vi "运维调试.vi"() -> ()   [LabVIEW 2016]
uses:
  <vilib>/Utility/miscctls.llb/LVPointTypeDef.ctl
  PLC/PLC.lvlib
  API/CodCr/CodCr.lvlib
  <vilib>/Utility/config.llb/NI_LVConfig.lvlib
panel:
  in  "运维调试菜单":T1(xcontrol)
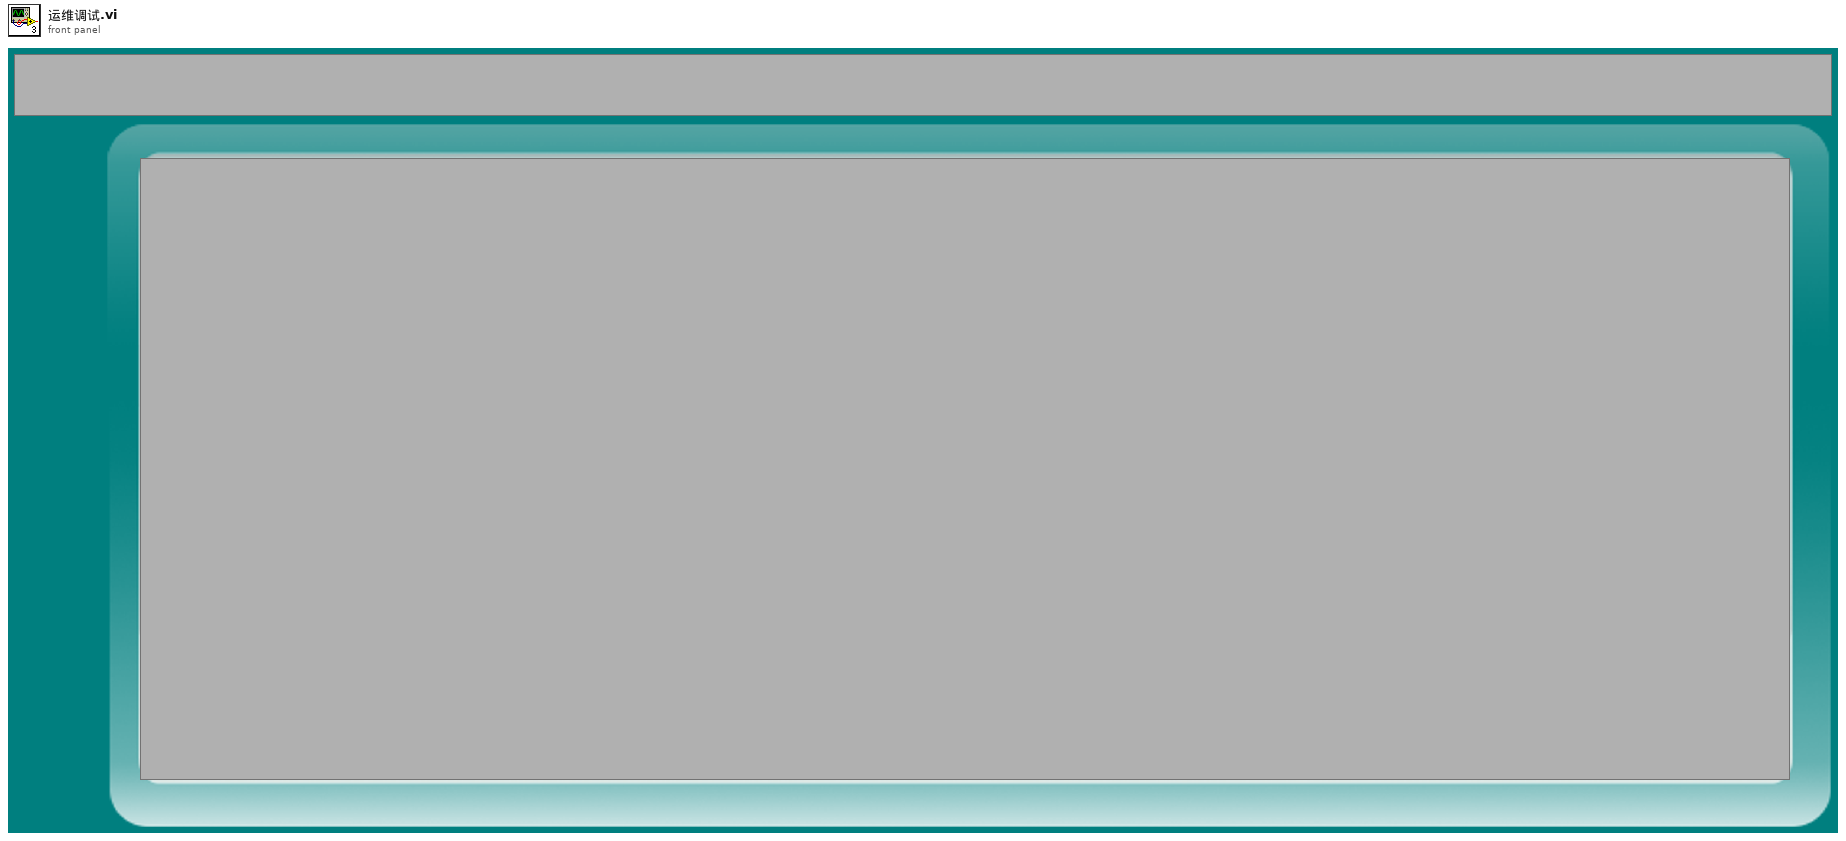
[diagram p1: front panel]
types:
  T1 = enum16{"电源管理", "采配水", "氨氮", "总磷", "总氮", "多参数", "CODMn", "CODcr", "流量计", "质控单元", "超标留样", "其他"}
  T2 = typedef "NI_LVConfig.lvlib/Config Data RefNum.ctl" = refnum<k1>
  T3 = typedef "LVPointTypeDef.ctl" = cluster{"Horizontal":i16, "Vertical":i16}
  T4 = enum16{"Enabled", "Disabled", "Disabled and Grayed Out"}
  T5 = enum32{"Bad", "Idle", "Run top level", "Running"}
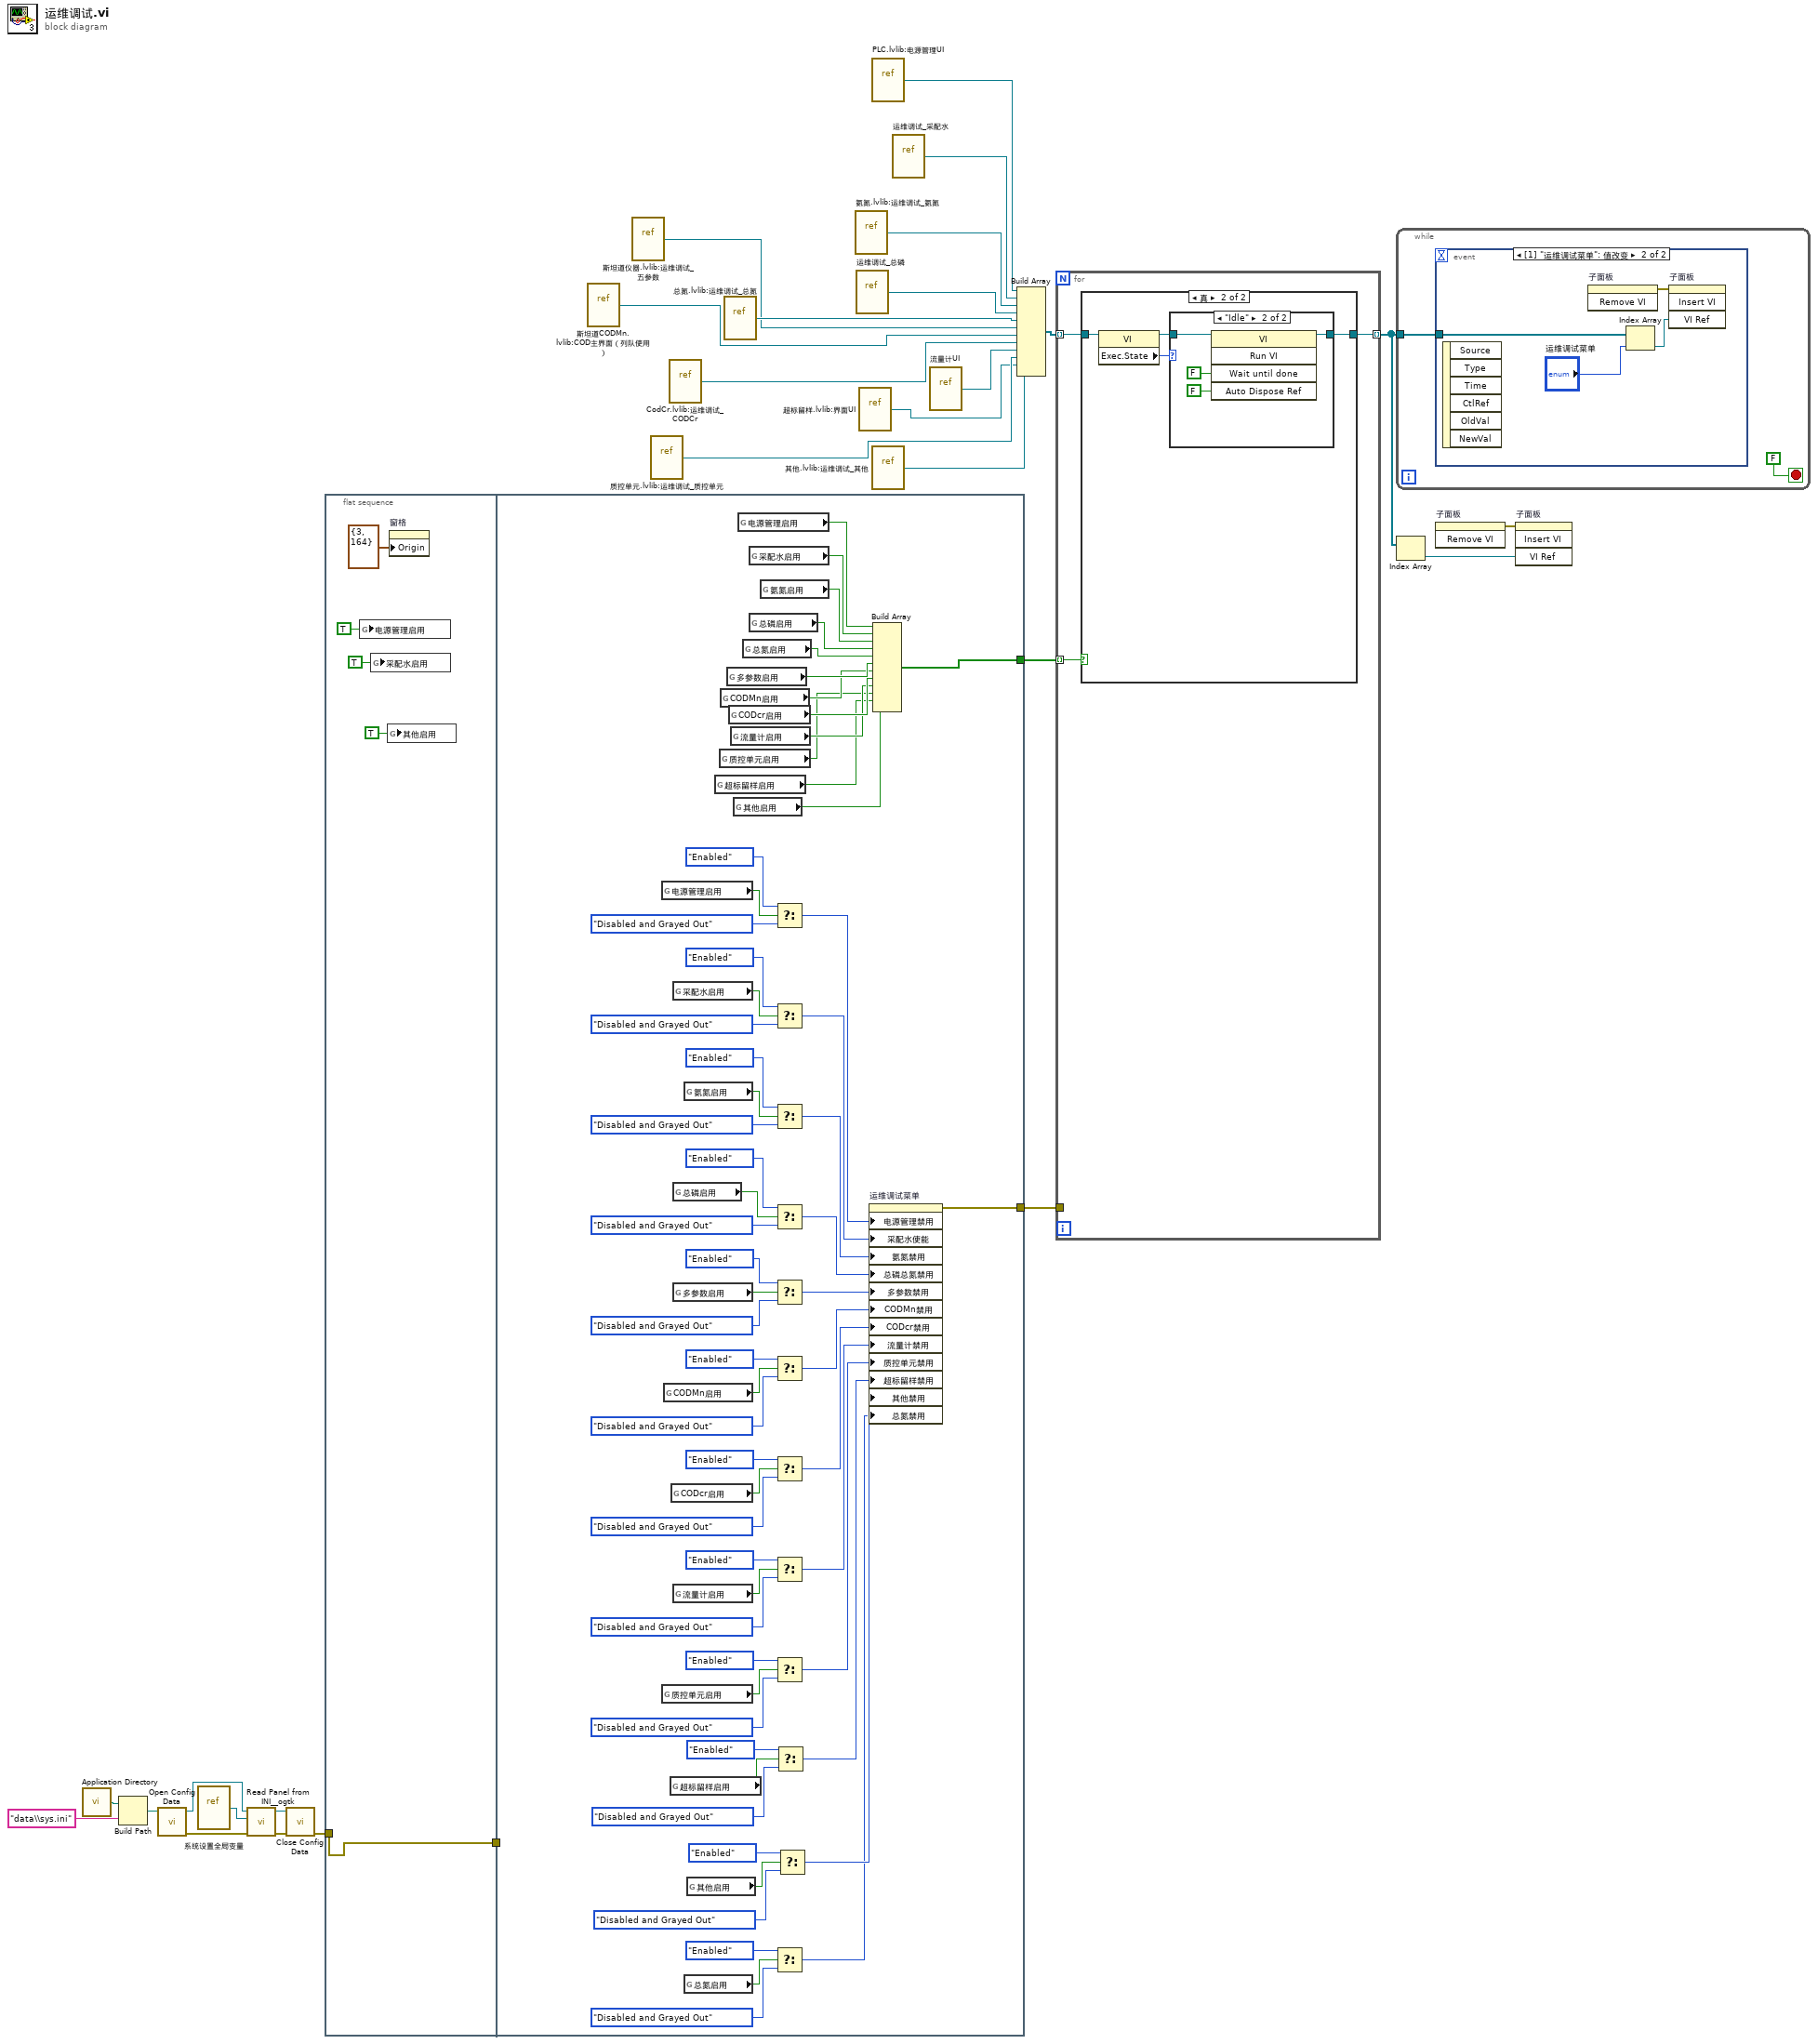
[diagram p0: block diagram]
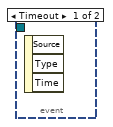
[diagram p4: hidden frame]
diagram:
  n1 = call <vilib>:"Application Directory.vi"() -> ("Application Directory"=w12:path)
  n2 = Build Path(base path=w12, name or relative path="data\\sys.ini" ("名称或相对路径")) -> (appended path=w10:path)
  n3 = call <vilib>:"Open Config Data.vi"("configuration file path"=w10) -> ("error out"=w19:errorcluster, "refnum"=w18:T2)  [unwired: 8 in, 1 out]
  n4 = vi-ref "系统设置全局变量.vi"() -> (w17:refnum<vi>)
  n5 = call <userlib>:"Read Panel from INI__ogtk.vi"("error in (no error)"=w19, "VI ref"=w17, "refnum"=w18) -> ("error out"=w16:errorcluster, "refnum out"=w15:T2)  [unwired: 7 in]
  n6 = call <vilib>:"Close Config Data.vi"("error in (no error)"=w16, "refnum"=w15) -> ("error out"=w14:errorcluster)  [unwired: 8 in, 1 out]
  n7 = flat-sequence {
    tunnel: w14 -> [w33]
    tunnel: [w33] -> w13
    tunnel: [w77] -> w20
    tunnel: w13 -> [_]
    tunnel: [w73] -> w9
    frame #0 {
      n8 = global write "系统设置全局变量.vi" "电源管理启用"(TRUE ("电源管理启用")) -> ()
      n9 = global write "系统设置全局变量.vi" "采配水启用"(TRUE ("采配水启用")) -> ()
      n10 = global write "系统设置全局变量.vi" "其他启用"(TRUE ("其他启用")) -> ()
      n11 = property on="窗格" class="Pane"("Origin"=T3 {"Horizontal"=3, "Vertical"=164} ("原点")) -> ()  [unwired: 2 in, 2 out]
    }
    frame #1 {
      n12 = global read "系统设置全局变量.vi" "电源管理启用"() -> (w95:bool)
      n13 = global read "系统设置全局变量.vi" "质控单元启用"() -> (w83:bool)
      n14 = global read "系统设置全局变量.vi" "CODMn启用"() -> (w86:bool)
      n15 = global read "系统设置全局变量.vi" "超标留样启用"() -> (w49:bool)
      n16 = global read "系统设置全局变量.vi" "CODcr启用"() -> (w85:bool)
      n17 = global read "系统设置全局变量.vi" "采配水启用"() -> (w92:bool)
      n18 = global read "系统设置全局变量.vi" "总磷启用"() -> (w34:bool)
      n19 = global read "系统设置全局变量.vi" "多参数启用"() -> (w88:bool)
      n20 = global read "系统设置全局变量.vi" "流量计启用"() -> (w84:bool)
      n21 = global read "系统设置全局变量.vi" "氨氮启用"() -> (w91:bool)
      n22 = global read "系统设置全局变量.vi" "总氮启用"() -> (w36:bool)
      n23 = global read "系统设置全局变量.vi" "其他启用"() -> (w82:bool)
      n24 = global read "系统设置全局变量.vi" "超标留样启用"() -> (w40:bool)
      n25 = global read "系统设置全局变量.vi" "质控单元启用"() -> (w41:bool)
      n26 = global read "系统设置全局变量.vi" "CODMn启用"() -> (w44:bool)
      n27 = global read "系统设置全局变量.vi" "多参数启用"() -> (w45:bool)
      n28 = global read "系统设置全局变量.vi" "CODcr启用"() -> (w43:bool)
      n29 = global read "系统设置全局变量.vi" "流量计启用"() -> (w42:bool)
      n30 = global read "系统设置全局变量.vi" "其他启用"() -> (w39:bool)
      n31 = global read "系统设置全局变量.vi" "电源管理启用"() -> (w74:bool)
      n32 = global read "系统设置全局变量.vi" "总氮启用"() -> (w46:bool)
      n33 = global read "系统设置全局变量.vi" "采配水启用"() -> (w75:bool)
      n34 = global read "系统设置全局变量.vi" "总磷启用"() -> (w47:bool)
      n35 = global read "系统设置全局变量.vi" "氨氮启用"() -> (w76:bool)
      n36 = Select(t=T4."Enabled" ("电源管理禁用"), s=w95, f=T4."Disabled and Grayed Out" ("电源管理禁用")) -> (s? t:f=w94:T4)
      n37 = Select(t=T4."Enabled" ("电源管理禁用"), s=w92, f=T4."Disabled and Grayed Out" ("电源管理禁用")) -> (s? t:f=w93:T4)
      n38 = Select(t=T4."Enabled" ("电源管理禁用"), s=w91, f=T4."Disabled and Grayed Out" ("电源管理禁用")) -> (s? t:f=w90:T4)
      n39 = Select(t=T4."Enabled" ("电源管理禁用"), s=w34, f=T4."Disabled and Grayed Out" ("电源管理禁用")) -> (s? t:f=w89:T4)
      n40 = Select(t=T4."Enabled" ("电源管理禁用"), s=w88, f=T4."Disabled and Grayed Out" ("电源管理禁用")) -> (s? t:f=w87:T4)
      n41 = Select(t=T4."Enabled" ("电源管理禁用"), s=w86, f=T4."Disabled and Grayed Out" ("电源管理禁用")) -> (s? t:f=w81:T4)
      n42 = Select(t=T4."Enabled" ("电源管理禁用"), s=w85, f=T4."Disabled and Grayed Out" ("电源管理禁用")) -> (s? t:f=w80:T4)
      n43 = Select(t=T4."Enabled" ("电源管理禁用"), s=w84, f=T4."Disabled and Grayed Out" ("电源管理禁用")) -> (s? t:f=w79:T4)
      n44 = Select(t=T4."Enabled" ("电源管理禁用"), s=w83, f=T4."Disabled and Grayed Out" ("电源管理禁用")) -> (s? t:f=w78:T4)
      n45 = Select(t=T4."Enabled" ("电源管理禁用"), s=w36, f=T4."Disabled and Grayed Out" ("电源管理禁用")) -> (s? t:f=w35:T4)
      n46 = Select(t=T4."Enabled" ("电源管理禁用"), s=w49, f=T4."Disabled and Grayed Out" ("电源管理禁用")) -> (s? t:f=w48:T4)
      n47 = Select(t=T4."Enabled" ("电源管理禁用"), s=w82, f=T4."Disabled and Grayed Out" ("电源管理禁用")) -> (s? t:f=w52:T4)
      n48 = property on="运维调试菜单" class="运维调试菜单 (严格)"("电源管理禁用"=w94, "采配水使能"=w93, "氨氮禁用"=w90, "总磷总氮禁用"=w89, "多参数禁用"=w87, "CODMn禁用"=w81, "CODcr禁用"=w80, "流量计禁用"=w79, "质控单元禁用"=w78, "超标留样禁用"=w48, "其他禁用"=w52, "总氮禁用"=w35) -> (error out=w77:errorcluster)  [unwired: 2 in, 1 out]
      n49 = Build Array(w74, w75, w76, w47, w46, w45, w44, w43, w42, w41, w40, w39) -> (w73:bool[])
    }
  }
  n50 = vi-ref "斯坦道CODMn.lvlib:COD主界面（列队使用）.vi"() -> (w6:refnum<vi>)
  n51 = vi-ref "斯坦道仪器.lvlib:运维调试_五参数.vi"() -> (w7:refnum<vi>)
  n52 = vi-ref "质控单元.lvlib:运维调试_质控单元.vi"() -> (w3:refnum<vi>)
  n53 = vi-ref "CodCr.lvlib:运维调试_CODCr.vi"() -> (w5:refnum<vi>)
  n54 = vi-ref "总氮.lvlib:运维调试_总氮.vi"() -> (w8:refnum<vi>)
  n55 = vi-ref "氨氮.lvlib:运维调试_氨氮.vi"() -> (w23:refnum<vi>)
  n56 = vi-ref "运维调试_总磷.vi"() -> (w22:refnum<vi>)
  n57 = vi-ref "超标留样.lvlib:界面UI.vi"() -> (w2:refnum<vi>)
  n58 = vi-ref "PLC.lvlib:电源管理UI.vi"() -> (w21:refnum<vi>)
  n59 = vi-ref "其他.lvlib:运维调试_其他.vi"() -> (w1:refnum<vi>)
  n60 = vi-ref "运维调试_采配水.vi"() -> (w24:refnum<vi>)
  n61 = vi-ref "流量计UI.vi"() -> (w4:refnum<vi>)
  n62 = Build Array(w21, w24, w23, w22, w8, w7, w6, w5, w4, w3, w2, w1) -> (w25:refnum<vi>[])
  n63 = for {
    tunnel: w25 -> [w98] mode=indexing
    tunnel: [w97] -> w27 mode=indexing
    tunnel: w9 -> [w96] mode=indexing
    tunnel: w20 -> [_]
    n64 = case shown="真" w96 {
      tunnel: w98 -> [w99 w103]
      tunnel: [w99 w100] -> w97
      frame False {
      }
      frame True {
        n65 = property class="VI"(reference=w103) -> (reference out=w101:refnum<vi>, "Exec.State"=w102:T5)  [unwired: 1 in, 1 out]
        n66 = case shown="\"Idle\"" w102 {
          tunnel: w101 -> [w104 w106]
          tunnel: [w104 w105] -> w100
          frame "Bad", Default {
          }
          frame "Idle" {
            n67 = invoke class="VI" method="Run VI"(reference=w106, "Wait until done"=FALSE ("结束前等待"), "Auto Dispose Ref"=FALSE ("自动销毁引用")) -> (reference out=w105:refnum<vi>)  [unwired: 2 in, 4 out]
          }
        }
      }
    }
  }
  n68 = while {
    tunnel: w27 -> [w109]
    stop <- FALSE stop-if-true
    n69 = event shown="[1] \"运维调试菜单\": 值改变" {
      selector: _ -> [_ _]
      dyn-events: _ -> [_ _]
      timeout: _ -> [_ _]
      tunnel: w109 -> [_ w113]
      event Timeout {
        n70 = event-data() -> ()  [unwired: 1 in, 3 out]
      }
      event "运维调试菜单": Value Change {
        n71 = event-data() -> ()  [unwired: 1 in, 6 out]
        n72 = invoke on="子面板" class="SubPnl" method="Remove VI"() -> (error out=w114:errorcluster)  [unwired: 3 in, 2 out]
        n73 = Index Array(array=w113, index="运维调试菜单") -> (element=w112:refnum<vi>)
        n74 = invoke on="子面板" class="SubPnl" method="Insert VI"(error in=w114, "VI Ref"=w112) -> ()  [unwired: 2 in, 4 out]
      }
    }
  }
  n75 = Index Array(array=w27) -> (element=w26:refnum<vi>)  [unwired: 1 in]
  n76 = invoke on="子面板" class="SubPnl" method="Remove VI"() -> (error out=w28:errorcluster)  [unwired: 3 in, 2 out]
  n77 = invoke on="子面板" class="SubPnl" method="Insert VI"(error in=w28, "VI Ref"=w26) -> ()  [unwired: 2 in, 4 out]
